vi "Visulaize.vi"() -> ()   [LabVIEW 2013, in "Phonocardiography.lvlib"]
uses:
  Phonocardiography.lvlib
  <vilib>/sound2/lvsound2.llb/Sampling Mode.ctl
  <vilib>/sound2/lvsound2.llb/Sound Data Format.ctl
  <vilib>/sound2/lvsound2.llb/Sound Input Read (DBL).vi
panel:
  in  "Samples per\nLoop":i32=8192
  in  "Device ID":u32
  out "Heart\nsound":waveform(dbl)(graph)
  in  "Stop":bool
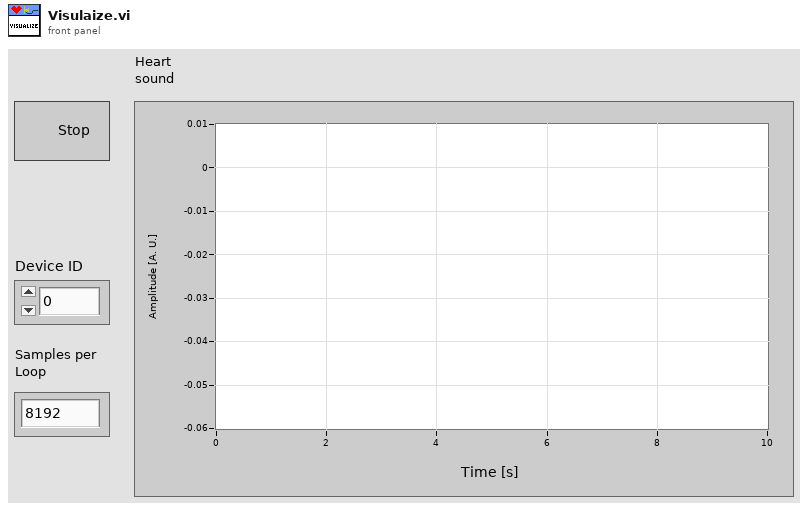
[diagram p1: front panel]
types:
  T1 = typedef "Sound Data Format.ctl" = cluster{"sample rate (S/s)":dbl, "number of channels":i32, "bits per sample":i32}
  T2 = typedef "Sampling Mode.ctl" = i32
  T3 = typedef "Sound Input Task ID.ctl" = u32
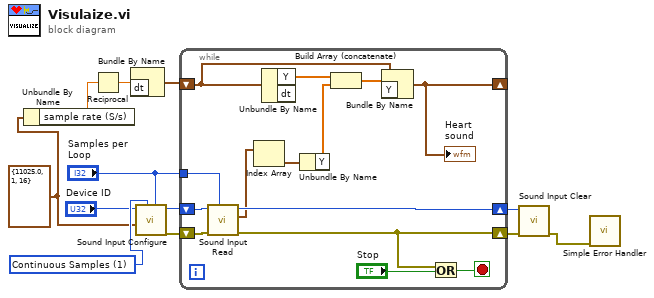
[diagram p0: block diagram]
diagram:
  w5 = T1 {"sample rate (S/s)"=11025.0, "number of channels"=1, "bits per sample"=16} ("Sound Format")
  w12 = T2 1 items=["Finite Samples", "Continuous Samples"] ("sample mode")
  n1 = Unbundle By Name(w5) -> ("sample rate (S/s)"=w2:dbl)
  n2 = Reciprocal(x=w2) -> (1/x=w4:dbl)
  n3 = Bundle By Name("dt"=w4) -> (w3:waveform(dbl))  [unwired: 1 in]
  n4 = call <vilib>:"Sound Input Configure.vi"("number of samples/ch"="Samples per\nLoop", "sample mode"=w12, "sound format"=w5, "device ID"="Device ID") -> ("error out"=w8:errorcluster, "task ID"=w9:T3)  [unwired: 6 in]
  n5 = while {
    tunnel: "Samples per\nLoop" -> [w23]
    shift-right: [w24] -> w10
    shift-left: w9 -> [w25]
    shift-right: [w13] -> w11
    shift-left: w8 -> [w26]
    shift-right: [w15] -> _
    shift-left: w3 -> [w17]
    stop <- w22 stop-if-true
    n6 = call-poly <vilib>:"Sound Input Read.vi"("number of samples/ch"=w23, "error in (no error)"=w26, "task ID"=w25) -> ("error out"=w13:errorcluster, "data"=w21:waveform(dbl)[], "task ID out"=w24:T3)  [unwired: 6 in]
    n7 = Index Array(array=w21) -> (element=w20:waveform(dbl))  [unwired: 1 in]
    n8 = Unbundle By Name(w17) -> ("Y"=w19:dbl[])  [unwired: 1 out]
    n9 = Unbundle By Name(w20) -> ("Y"=w18:dbl[])
    n10 = Build Array (concatenate)(w19, w18) -> (w16:dbl[])
    n11 = Bundle By Name(cluster=w17, "Y"=w16) -> (w15:waveform(dbl))
    "Heart\nsound" <- w15
    n12 = Or(x=w13, y="Stop") -> (x .or. y?=w22:bool)
  }
  n13 = call <vilib>:"Sound Input Clear.vi"("error in (no error)"=w11, "task ID"=w10) -> ("error out"=w1:errorcluster)  [unwired: 9 in]
  n14 = call <vilib>:"Simple Error Handler.vi"("error in (no error)"=w1) -> ()  [unwired: 4 in, 5 out]
